vi "Dropout.vi"(7 "Droput Prob":dbl, 9 "Biases":dbl[](array[numeric]), 10 "Weights":dbl[][](array[numeric]), 11 "Data":dbl[](array[numeric])) -> (1 "Droupout Biases":dbl[](array[numeric]), 2 "Dropout Weights":dbl[][](array[numeric]), 3 "Droput Data":dbl[](array[numeric]))   [LabVIEW 2020]
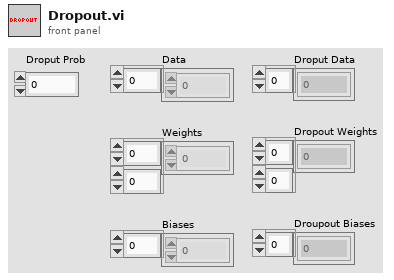
[diagram p1: front panel]
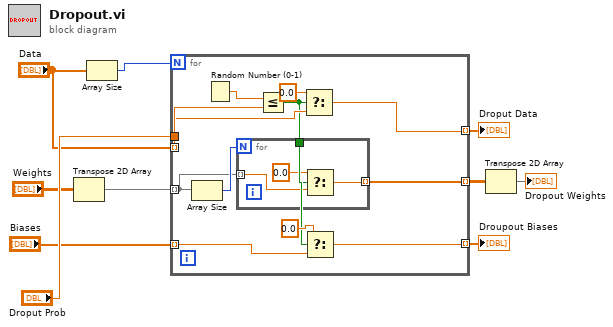
[diagram p0: block diagram]
diagram:
  n1 = Transpose 2D Array(2D array="Weights") -> (transposed array=w4:dbl[][])
  n2 = Array Size(array="Data") -> (size(s)=w10:i32)
  n3 = for {
    N: w10 -> [_]
    tunnel: "Droput Prob" -> [w21]
    tunnel: "Data" -> [w20] mode=indexing
    tunnel: [w18] -> w7 mode=indexing
    tunnel: "Biases" -> [w16] mode=indexing
    tunnel: w4 -> [w11] mode=indexing
    tunnel: [w14] -> w3 mode=indexing
    tunnel: [w12] -> w1 mode=indexing
    n4 = Array Size(array=w11) -> (size(s)=w13:i32)
    n5 = Random Number (0-1)() -> (number: 0 to 1=w22:dbl)
    n6 = Less Or Equal?(x=w22, y=w21) -> (x <= y?=w15:bool)
    n7 = for {
      N: w13 -> [_]
      tunnel: w15 -> [w26]
      tunnel: [w24] -> w14 mode=indexing
      tunnel: w11 -> [w23] mode=indexing
      n8 = Select(t=0.0, s=w26, f=w23) -> (s? t:f=w24:dbl)
    }
    n9 = Select(t=0.0, s=w15, f=w20) -> (s? t:f=w18:dbl)
    n10 = Select(t=0.0, s=w15, f=w16) -> (s? t:f=w12:dbl)
  }
  "Droput Data" <- w7
  "Droupout Biases" <- w1
  n11 = Transpose 2D Array(2D array=w3) -> (transposed array=→"Dropout Weights":dbl[][])
